vi "בדיקת צריכת זרם של סליל הפיקוד 4.vi"(7 "resultUserPrompt":bool, 8 "error":errorcluster, 11 "Path for Log":path) -> (0 "error out":errorcluster, 2 "צריכת זרם בסליל בטווח כן/לא":bool, 3 "צריכת זרם בסליל":dbl format="%.4f")   [LabVIEW 2014]
uses:
  <vilib>/DAQmx/create/channels.llb/DAQmx Create Channel (DO-Digital Output).vi
  <vilib>/DAQmx/write.llb/DAQmx Write (Digital Bool 1Line 1Point).vi
panel:
  # "Right-Click to\nexplain error"
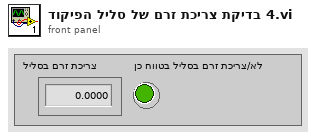
[diagram p1: front panel]
types:
  T1 = enum32{"Invalid", "Standard", "Closed", "Hidden", "Minimized", "Maximized"}
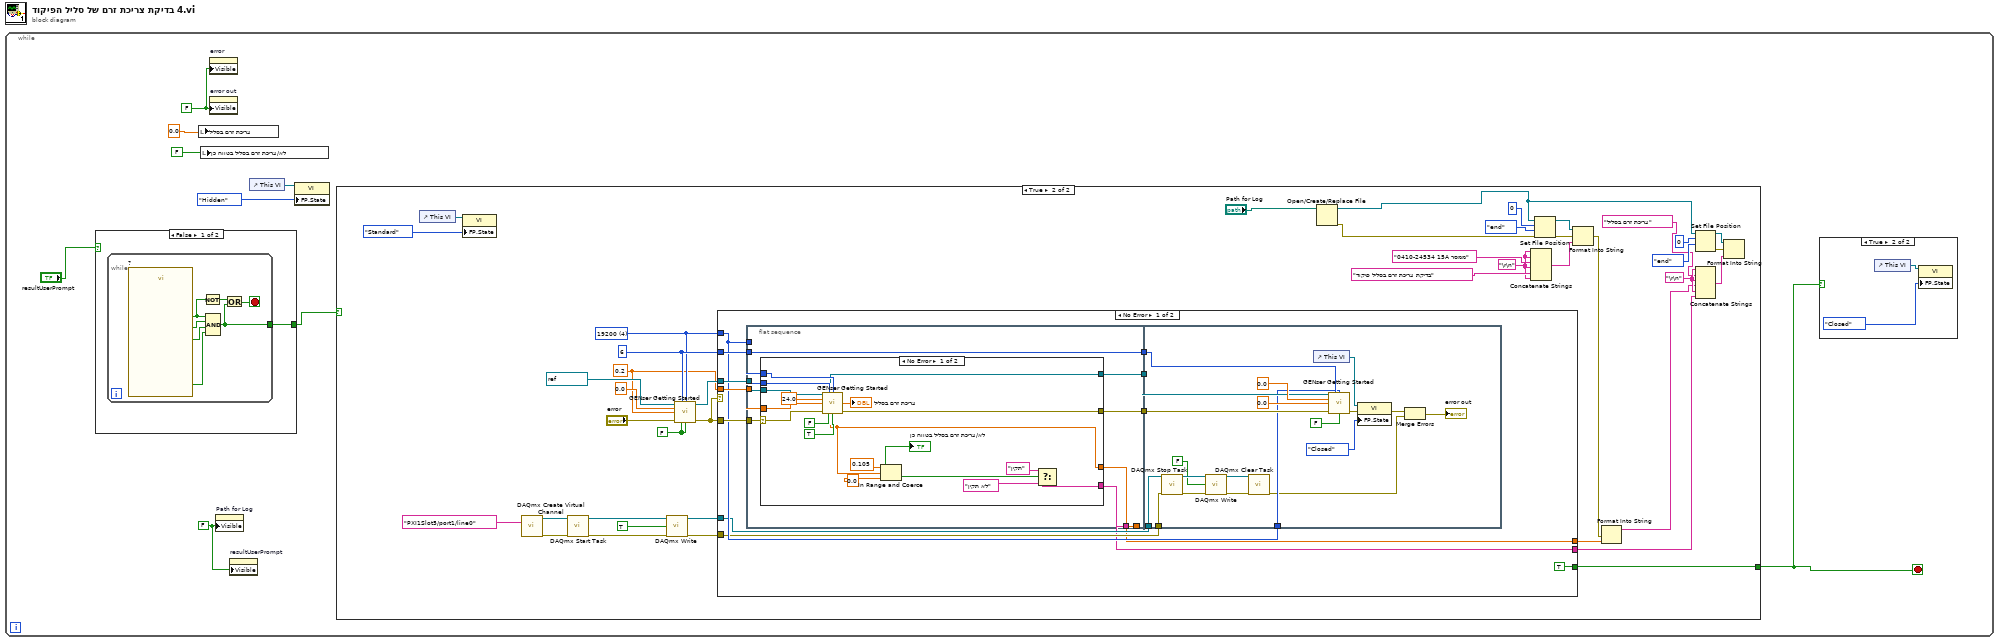
[diagram p0: block diagram]
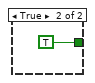
[diagram p3: hidden frame]
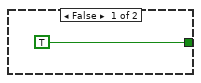
[diagram p4: hidden frame]
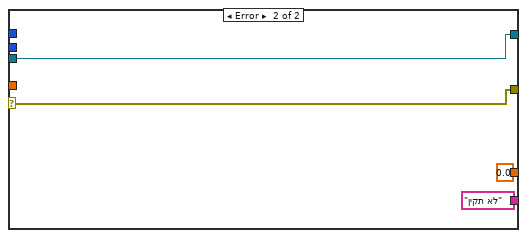
[diagram p5: hidden frame]
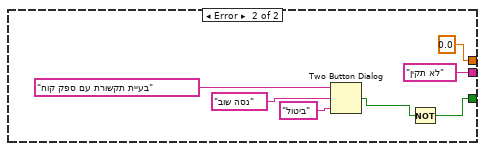
[diagram p6: hidden frame]
diagram:
  n1 = while {
    stop <- w1 stop-if-true
    w2 = FALSE ("Visible")
    w6 = FALSE ("Visible")
    n2 = case shown="False" "resultUserPrompt" {
      tunnel: [w12 TRUE] -> w9
      frame False {
        n3 = while {
          tunnel: [w13] -> w12
          stop <- w16 stop-if-true
          n4 = call "?"() -> ("הדקי הרב מודד"=w17:bool, "(מגע שלילי (מעטפת"=w18:bool, "A מגע חיובי"=w19:bool, "OK"=w14:bool)  [unwired: 15 in, 1 out]
          n5 = Not(x=w14) -> (.not. x?=w15:bool)
          n6 = Compound Arithmetic op=AND(w14, w19, w18, w17) -> (w13:bool)
          n7 = Or(x=w15, y=w13) -> (x .or. y?=w16:bool)
        }
      }
      frame True {
      }
    }
    n8 = local write "צריכת זרם בסליל"(0.0 ("Output Current")) -> ()
    n9 = local write "צריכת זרם בסליל בטווח כן/לא"(FALSE ("In Range?")) -> ()
    n10 = property on="error" class="Clust (strict)"("Visible"=w6) -> ()  [unwired: 2 in, 2 out]
    n11 = property on="error out" class="Clust (strict)"("Visible"=w6) -> ()  [unwired: 2 in, 2 out]
    n12 = property on="Path for Log" class="Path"("Visible"=w2) -> ()  [unwired: 2 in, 2 out]
    n13 = property on="resultUserPrompt" class="Bool (strict)"("Visible"=w2) -> ()  [unwired: 2 in, 2 out]
    n14 = control-ref of="This VI"() -> (w5:refnum<vi>)
    n15 = property class="VI"(reference=w5, "FP.State"=T1."Hidden" ("Front Panel Window:State")) -> ()  [unwired: 1 in, 2 out]
    n16 = case shown="True" w9 {
      tunnel: [TRUE ("T button?") w55] -> w1
      frame False {
      }
      frame True {
        w28 = "\r\n"
        w37 = "\r\n"
        w54 = FALSE ("Output On (T)")
        w59 = u16 4 items=["1200", "2400", "4800", "9600", "19200"] ("BAUD")
        w60 = i16 6 ("GEN Addr")
        w56 = 0.2 ("Current Limit")
        n17 = control-ref of="This VI"() -> (w53:refnum<vi>)
        n18 = property class="VI"(reference=w53, "FP.State"=T1."Standard" ("Front Panel Window:State")) -> ()  [unwired: 1 in, 2 out]
        n19 = call-poly <vilib>:"DAQmx Create Virtual Channel.vi"("lines"=tag "PXI1Slot5/port1/line0") -> ("task out"=w50:refnum<k21>, "error out"=w51:errorcluster)  [unwired: 13 in]
        n20 = call <vilib>:"DAQmx Start Task.vi"("task/channels in"=w50, "error in"=w51) -> ("task out"=w48:refnum<k21>, "error out"=w47:errorcluster)  [unwired: 12 in]
        n21 = call-poly <vilib>:"DAQmx Write.vi"("task/channels in"=w48, "data"=TRUE, "error in"=w47) -> ("task out"=w45:refnum<k21>, "error out"=w44:errorcluster)  [unwired: 10 in, 1 out]
        n22 = call "GENser Getting Started.vi"("VISA"=refnum<visa-resource-name> "COM6", "GEN Addr"=w60, "BAUD"=w59, "Voltage Limit"=0.0, "Current Limit"=w56, "error"="error", "Reset (T)"=w54, "Output On (T)"=w54) -> ("VISA out"=w61:refnum<visa-resource-name>, "error out"=w62:errorcluster)  [unwired: 4 in, 2 out]
        n23 = case shown="No Error" w62 {
          tunnel: w62 -> [w71 _]
          tunnel: w61 -> [w73 _]
          tunnel: w60 -> [w74 _]
          tunnel: w59 -> [w68 _]
          tunnel: w56 -> [w72 _]
          tunnel: [TRUE w127] -> w55
          tunnel: w45 -> [w67 _]
          tunnel: w44 -> [w66 _]
          tunnel: [w65 0.0 ("Output Current")] -> w34
          tunnel: [w64 "לא תקין"] -> w26
          frame No Error {
            n24 = flat-sequence {
              tunnel: [w85] -> w75
              tunnel: w68 -> [w84]
              tunnel: w74 -> [w80]
              tunnel: w73 -> [w83]
              tunnel: w72 -> [w82]
              tunnel: w71 -> [w79]
              tunnel: [w81] -> w70
              tunnel: [w80] -> w69
              tunnel: [w78] -> w65
              tunnel: [w77] -> w64
              tunnel: w75 -> [w123]
              tunnel: w70 -> [w122]
              tunnel: w69 -> [w121]
              tunnel: w68 -> [w120]
              tunnel: w67 -> [w108]
              tunnel: w66 -> [w107]
              frame #0 {
                n25 = case shown="No Error" w79 {
                  selector: w79 -> [w91 w105]
                  tunnel: [w97 w105] -> w85
                  tunnel: w84 -> [w96 _]
                  tunnel: w80 -> [w95 _]
                  tunnel: w83 -> [w94 w106]
                  tunnel: w82 -> [w93 _]
                  tunnel: [w92 w106] -> w81
                  tunnel: [w90 0.0 ("Output Current")] -> w78
                  tunnel: [w86 "לא תקין"] -> w77
                  frame No Error {
                    n26 = call "GENser Getting Started.vi"("VISA"=w94, "GEN Addr"=w95, "BAUD"=w96, "Voltage Limit"=24.0, "Current Limit"=w93, "error"=w91, "Reset (T)"=FALSE, "Output On (T)"=TRUE) -> ("VISA out"=w92:refnum<visa-resource-name>, "Output Current"=w90:dbl, "error out"=w97:errorcluster)  [unwired: 4 in, 1 out]
                    "צריכת זרם בסליל" <- w90
                    n27 = In Range and Coerce(upper limit=0.105, x=w90, lower limit=0.0) -> (In Range?=w87:bool)  [unwired: 1 out]
                    "צריכת זרם בסליל בטווח כן/לא" <- w87
                    n28 = Select(t="תקין", s=w87, f="לא תקין") -> (s? t:f=w86:string)
                  }
                  frame Error {
                  }
                }
              }
              frame #1 {
                n29 = call <vilib>:"DAQmx Stop Task.vi"("task/channels in"=w108, "error in"=w107) -> ("task out"=w116:refnum<k21>, "error out"=w115:errorcluster)  [unwired: 12 in]
                n30 = call-poly <vilib>:"DAQmx Write.vi"("task/channels in"=w116, "data"=FALSE, "error in"=w115) -> ("task out"=w114:refnum<k21>, "error out"=w113:errorcluster)  [unwired: 10 in, 1 out]
                n31 = call <vilib>:"DAQmx Clear Task.vi"("task in"=w114, "error in"=w113) -> ("error out"=w110:errorcluster)  [unwired: 13 in]
                n32 = control-ref of="This VI"() -> (w119:refnum<vi>)
                n33 = call "GENser Getting Started.vi"("VISA"=w122, "GEN Addr"=w121, "BAUD"=w120, "Voltage Limit"=0.0, "Current Limit"=0.0, "error"=w123, "Output On (T)"=FALSE) -> ("error out"=w117:errorcluster)  [unwired: 5 in, 3 out]
                n34 = property class="VI"(reference=w119, error in=w117, "FP.State"=T1."Closed" ("Front Panel Window:State")) -> (error out=w111:errorcluster)  [unwired: 1 out]
                n35 = Merge Errors(w111, w110) -> (→"error out":errorcluster)
              }
            }
          }
          frame Error {
            n36 = Two Button Dialog(message="בעיית תקשורת עם ספק קוח", 1:"ביטול" ("F button name (\"Cancel\")"), 2:"נסה שוב" ("T button name (\"OK\")")) -> (T button?=w128:bool)
            n37 = Not(x=w128) -> (.not. x?=w127:bool)
          }
        }
        n38 = Open/Create/Replace File(file path (use dialog)="Path for Log") -> (refnum out=w22:refnum<file>, error out=w23:errorcluster)  [unwired: 5 in, 1 out]
        n39 = Concatenate Strings(w37, w37, "0410-24534 15A ממסר", w37, "בדיקת צריכת זרם בסליל פיקוד", w37) -> (w41:string)
        n40 = Set File Position(offset (in bytes) (0)=i64 0, refnum=w22, from (0:start)=enum16{"start", "end", "current"}."end", error in=w23) -> (refnum out=w38:refnum<file>, error out=w36:errorcluster)
        n41 = Format Into String(initial string=w38, error in=w36, w41) -> (error out=w35:errorcluster)  [unwired: 1 in, 1 out]
        n42 = Format Into String(error in=w35, w34) -> (resulting string=w25:string)  [unwired: 2 in, 1 out]
        n43 = Set File Position(offset (in bytes) (0)=i64 0, refnum=w22, from (0:start)=enum16{"start", "end", "current"}."end") -> (refnum out=w31:refnum<file>, error out=w32:errorcluster)  [unwired: 1 in]
        n44 = Concatenate Strings(w28, "צריכת זרם בסליל", w28, w25, w28, w26) -> (w33:string)
        n45 = Format Into String(initial string=w31, error in=w32, w33) -> ()  [unwired: 1 in, 2 out]
      }
    }
    n46 = case shown="True" w1 {
      frame False {
      }
      frame True {
        n47 = control-ref of="This VI"() -> (w10:refnum<vi>)
        n48 = property class="VI"(reference=w10, "FP.State"=T1."Closed" ("Front Panel Window:State")) -> ()  [unwired: 1 in, 2 out]
      }
    }
  }
